vi "main.vi"() -> ()   [LabVIEW 2024]
uses:
  Controls/#typedef_program_data_INFO.ctl
  Controls/#typedef_program_states.ctl
panel:
  out "error out":errorcluster
  in  "error in (no error)":errorcluster
  out "Info":T1={"Result"=TRUE, "Message"="", "Last contamination [%]"=0.0, "Attempts to clean"=0.0} {"Last contamination [%]" format="%#_3f"}
  in  "Stop":bool
  in  "Run cleaning":bool
  in  "Info IN":T1 {"Last contamination [%]" format="%#_3f"}
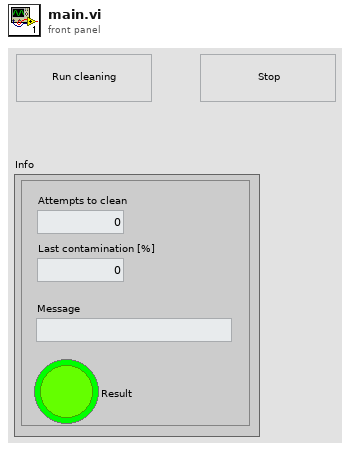
[diagram p1: front panel]
types:
  T1 = typedef "#typedef_program_data_INFO.ctl" = cluster{"Result":bool, "Message":string, "Last contamination [%]":dbl, "Attempts to clean":dbl}
  T2 = typedef "#typedef_program_states.ctl" = enum16{"application error", "init", "idle", "oczyszczanie", "sprawdzenie", "stop"}
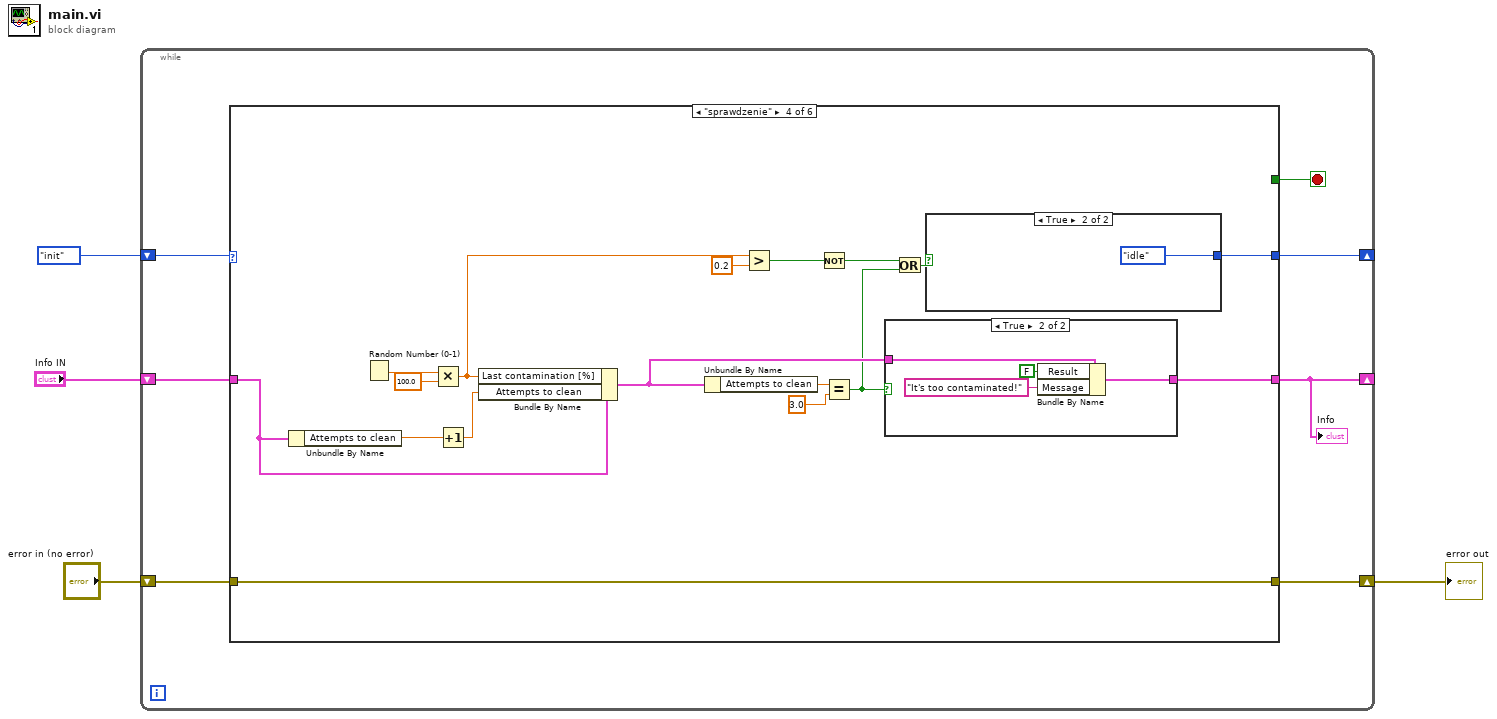
[diagram p0: block diagram]
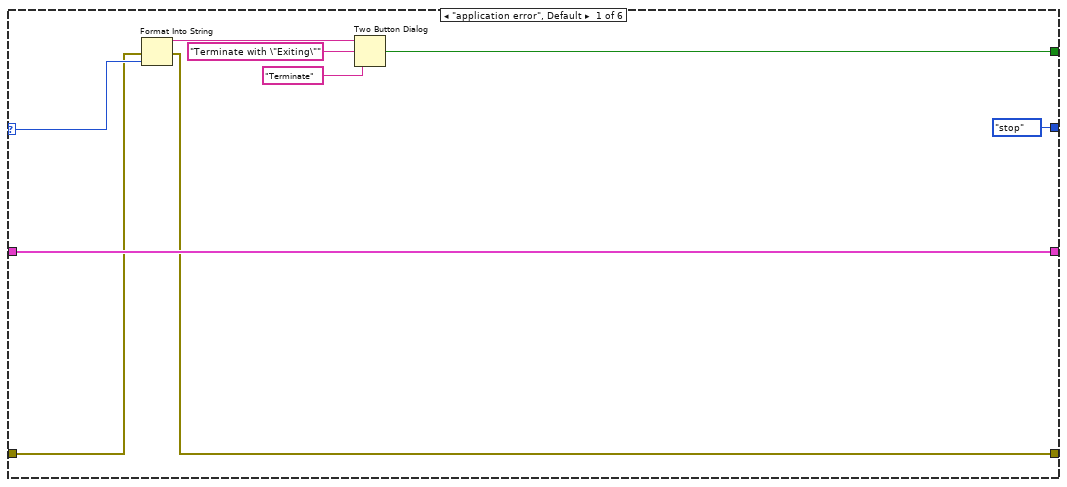
[diagram p2: hidden frame]
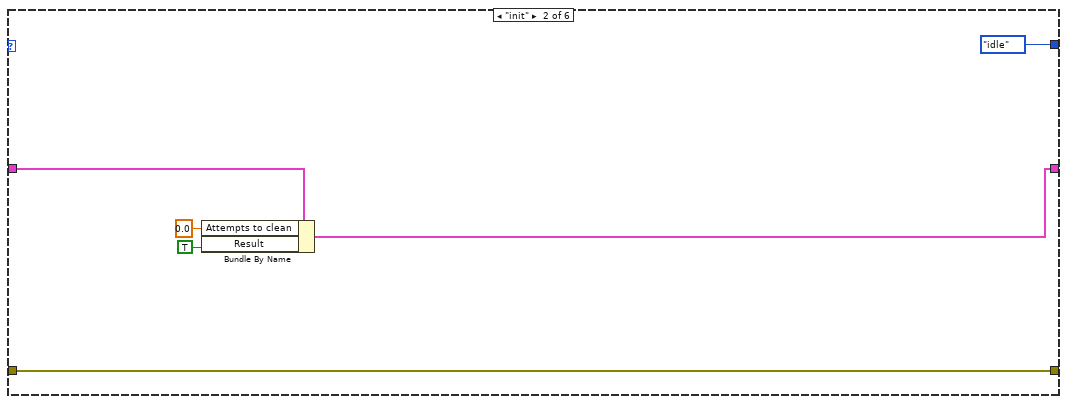
[diagram p3: hidden frame]
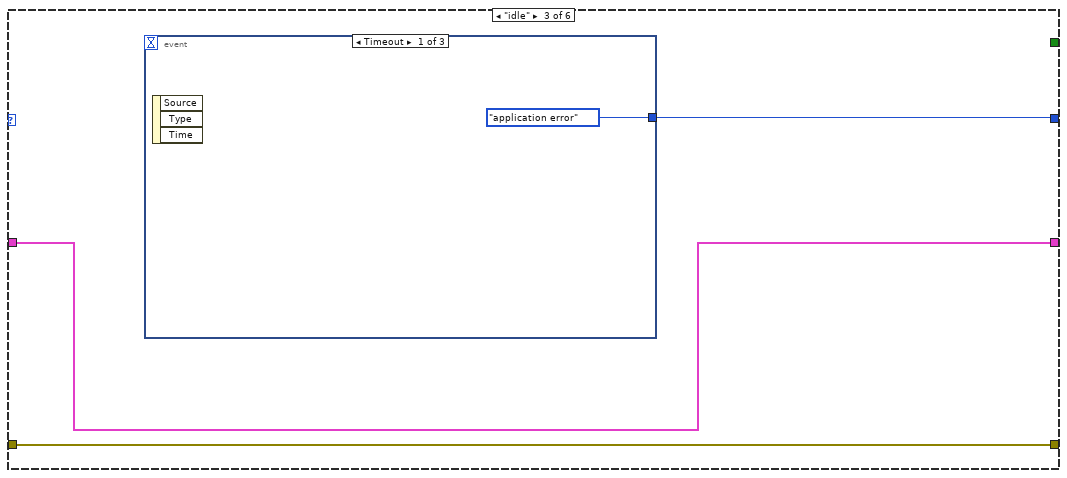
[diagram p4: hidden frame]
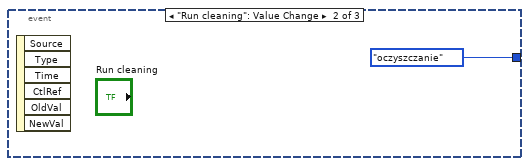
[diagram p5: hidden frame]
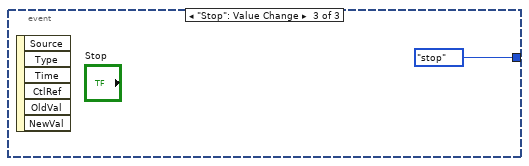
[diagram p6: hidden frame]
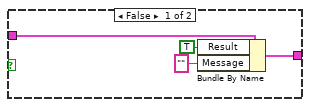
[diagram p7: hidden frame]
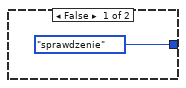
[diagram p8: hidden frame]
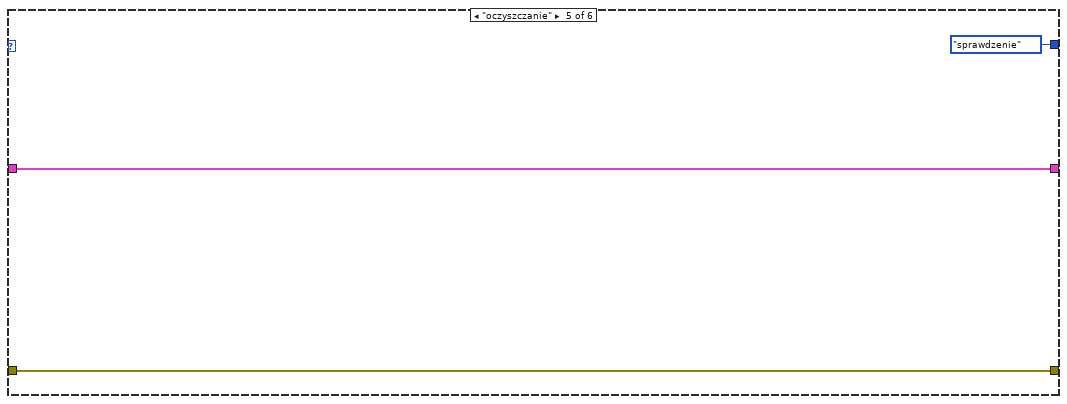
[diagram p9: hidden frame]
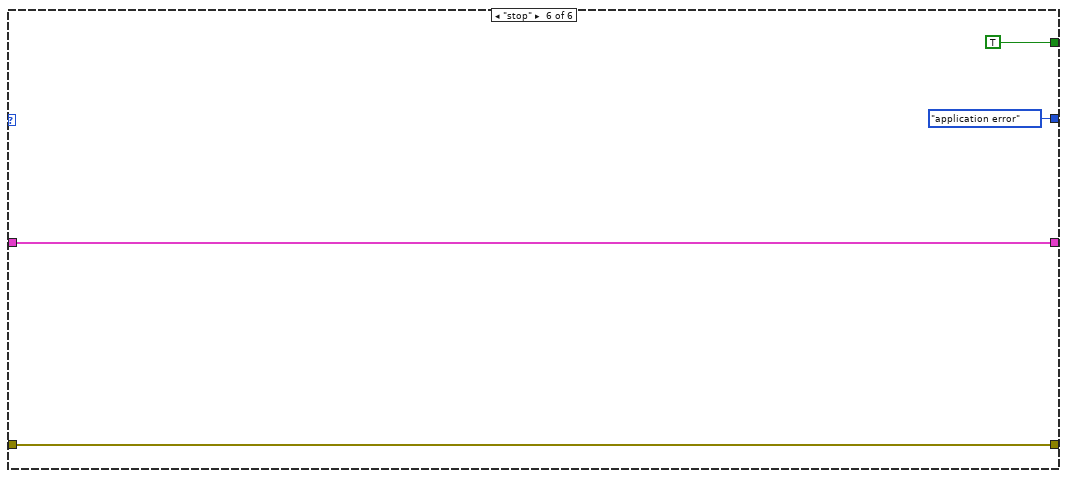
[diagram p10: hidden frame]
diagram:
  n1 = while {
    shift-right: [w10] -> _
    shift-left: #typedef_program_states."init" ("Program States") -> [w11]
    shift-right: [w7] -> _
    shift-left: "Info IN" -> [w8]
    shift-right: [w5] -> w1
    shift-left: "error in (no error)" -> [w6]
    stop <- w9 stop-if-true
    n2 = case shown="\"sprawdzenie\"" w11 {
      selector: w11 -> [w19 _ _ _ _ _]
      tunnel: [#typedef_program_states."stop" ("Program States") #typedef_program_states."idle" ("Program States") w29 w44 #typedef_program_states."sprawdzenie" ("Program States") #typedef_program_states."application error" ("Program States")] -> w10
      tunnel: [w15 _ _ _ _ TRUE] -> w9
      tunnel: w8 -> [w14 w25 w28 w43 w61 w64]
      tunnel: [w14 w23 w28 w37 w61 w64] -> w7
      tunnel: w6 -> [w13 w21 w27 w33 w60 w63]
      tunnel: [w12 w21 w27 w33 w60 w63] -> w5
      frame "application error", Default {
        n3 = Format Into String(error in=w13, w19) -> (resulting string=w18:string, error out=w12:errorcluster)  [unwired: 2 in]
        n4 = Two Button Dialog(message=w18, 1:"Terminate" ("F button name (\"Cancel\")"), 2:"Terminate with \"Exiting\"" ("T button name (\"OK\")")) -> (T button?=w15:bool)
      }
      frame "init" {
        n5 = Bundle By Name(cluster=w25, "Attempts to clean"=0.0, "Result"=TRUE) -> (w23:T1)
      }
      frame "idle" {
        n6 = event shown="[0] Timeout" {
          selector: _ -> [_ _ _]
          dyn-events: _ -> [_ _ _]
          timeout: _ -> [_ _ _]
          tunnel: [#typedef_program_states."application error" ("Program States") #typedef_program_states."oczyszczanie" ("Program States") #typedef_program_states."stop" ("Program States")] -> w29
          event Timeout {
            n7 = event-data() -> ()  [unwired: 1 in, 3 out]
          }
          event "Run cleaning": Value Change {
            n8 = event-data() -> ()  [unwired: 1 in, 6 out]
          }
          event "Stop": Value Change {
            n9 = event-data() -> ()  [unwired: 1 in, 6 out]
          }
        }
      }
      frame "sprawdzenie" {
        n10 = Unbundle By Name(w43) -> ("Attempts to clean"=w42:dbl)
        n11 = Random Number (0-1)() -> (number: 0 to 1=w49:dbl)
        n12 = Multiply(x=w49, y=100.0) -> (x*y=w47:dbl)
        n13 = Increment(x=w42) -> (x+1=w41:dbl)
        n14 = Bundle By Name(cluster=w43, "Last contamination [%]"=w47, "Attempts to clean"=w41) -> (w38:T1)
        n15 = Unbundle By Name(w38) -> ("Attempts to clean"=w40:dbl)
        n16 = Greater?(x=w47, y=0.2) -> (0:w45:bool)
        n17 = Not(x=w45) -> (.not. x?=w34:bool)
        n18 = Equal?(x=w40, y=3.0) -> (x = y?=w35:bool)
        n19 = case shown="True" w35 {
          tunnel: [w51 w57] -> w37
          tunnel: w38 -> [w50 w56]
          frame False {
            n20 = Bundle By Name(cluster=w50, "Result"=TRUE, "Message"="") -> (w51:T1)
          }
          frame True {
            n21 = Bundle By Name(cluster=w56, "Result"=FALSE, "Message"="It's too contaminated!") -> (w57:T1)
          }
        }
        n22 = Or(x=w34, y=w35) -> (x .or. y?=w36:bool)
        n23 = case shown="True" w36 {
          tunnel: [#typedef_program_states."sprawdzenie" ("Program States") #typedef_program_states."idle" ("Program States")] -> w44
          frame False {
          }
          frame True {
          }
        }
      }
      frame "oczyszczanie" {
      }
      frame "stop" {
      }
    }
    "Info" <- w7
  }
  "error out" <- w1
